vi "Multiple inputs.vi"() -> ()   [LabVIEW 2015]
doc: "This example VI shows how to convert string data elements to numeric elements so it can be graphed and displayed on an XY Graph."
uses:
  <instrlib>/Keithley 27XX/Keithley 27XX.lvlib
panel:
  in  "Column headers":string[](array[string])=["Time/s", "TH/Celsius", "TC/Celsius", "Delta V"]
  in  "Number of channels":i32=1
  in  "Pause/Continue":bool
  in  "stop":bool
  out "Numeric":i32
  out "concatenated string":string
  in  "file (use dialog)":path=path "C:/Users/Guest_2/Desktop/Zong Long/Data trial.txt"
  in  "Function (6: Temp)":u16(ring)=6 items=["DC Voltage", "AC Voltage", "DC Current", "AC Current", "Resistance", "Four-Wire Resistance", "Temperature (C)", "Frequency", "Period", "Continuity"]
  in  "Channel List (101)":string="101"
  in  "Serial Configuration":T1={"Baud Rate (9600)"=9600, "Flow Control (1: XON/XOFF)"=1, "Termination Char (0:CR)"=0} {"Termination Char (0:CR)" items=["CR", "LF", "CRLF (Do not use)", "LFCR (Do not use)"]; "Flow Control (1: XON/XOFF)" items=["None", "XON/XOFF", "RTS/CTS (2701 Only)", "XON/XOFF & RTS/CTS (2701 Only)"]; "Baud Rate (9600)" items=["300"=300, "600"=600, "1200"=1200, "2400"=2400, "4800"=4800, "9600"=9600, "19.2k"=19200, "38.4k (2701 Only)"=38400, "57.6k (2701 Only)"=57600, "115.2k (2701 Only)"=115200]}
  in  "VISA resource name":refnum<visa-resource-name>="GPIB0::19::INSTR"
  # "Remember to change the number of channels"
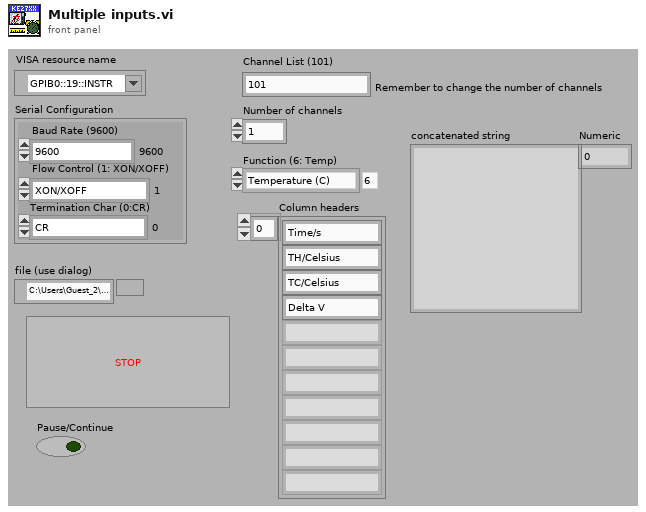
[diagram p1: front panel]
types:
  T1 = cluster{"Baud Rate (9600)":u32, "Flow Control (1: XON/XOFF)":u16, "Termination Char (0:CR)":u16}
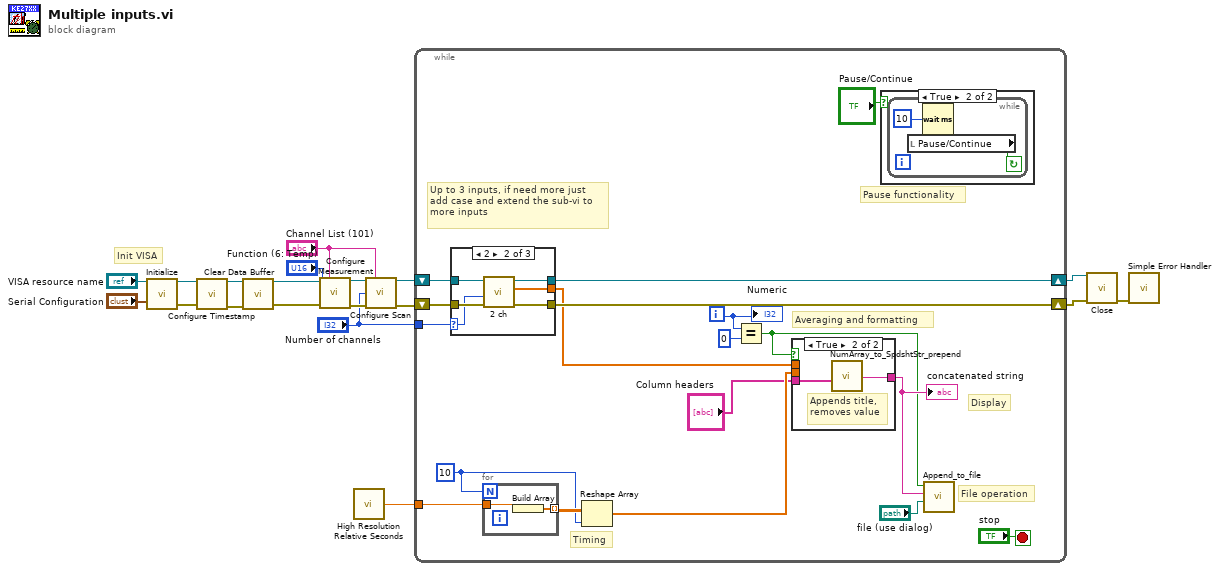
[diagram p0: block diagram]
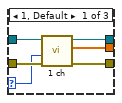
[diagram p2: hidden frame]
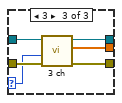
[diagram p3: hidden frame]
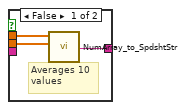
[diagram p5: hidden frame]
diagram:
  # "Init VISA"
  n1 = call <instrlib>:"Initialize.vi"("VISA resource name"="VISA resource name", "Serial Configuration"="Serial Configuration") -> ("VISA resource name out"=w16:refnum<visa-resource-name>, "error out"=w15:errorcluster)  [unwired: 12 in]
  n2 = call <instrlib>:"Configure Timestamp.vi"("VISA resource name"=w16, "error in (no error)"=w15) -> ("VISA resource name out"=w11:refnum<visa-resource-name>, "error out"=w10:errorcluster)  [unwired: 12 in]
  n3 = call <instrlib>:"Clear Data Buffer.vi"("VISA resource name"=w11, "error in (no error)"=w10) -> ("VISA resource name out"=w9:refnum<visa-resource-name>, "error out"=w12:errorcluster)  [unwired: 12 in]
  n4 = call <instrlib>:"Configure Measurement.vi"("VISA resource name"=w9, "Scan List (Empty)"="Channel List (101)", "Function (0: DC Voltage)"="Function (6: Temp)", "error in (no error)"=w12) -> ("VISA resource name out"=w8:refnum<visa-resource-name>, "error out"=w6:errorcluster)  [unwired: 10 in]
  n5 = call <vilib>:"High Resolution Relative Seconds.vi"() -> ("relative seconds"=w2:dbl)
  n6 = call <instrlib>:"Configure Scan.vi"("VISA resource name"=w8, "Channel List (101:110)"="Channel List (101)", "Sample Count (100)"="Number of channels", "error in (no error)"=w6) -> ("VISA resource name out"=w4:refnum<visa-resource-name>, "error out"=w3:errorcluster)  [unwired: 10 in]
  n7 = while {
    shift-right: [w36] -> w13
    shift-left: w4 -> [w35]
    shift-right: [w37] -> w14
    shift-left: w3 -> [w34]
    tunnel: w2 -> [w30]
    tunnel: "Number of channels" -> [w21]
    i -> [w24]
    stop <- "stop" stop-if-true
    w20 = 10 ("x")
    # "Timing"
    # "Up to 3 inputs, if need more just\nadd case and extend the sub-vi to\nmore inputs"
    # "Display"
    # "Averaging and formatting"
    # "File operation"
    # "Pause functionality"
    n8 = case shown="2" w21 {
      selector: w21 -> [w38 w44 w50]
      tunnel: [w41 w45 w51] -> w37
      tunnel: [w39 w47 w53] -> w36
      tunnel: w35 -> [w43 w49 w54]
      tunnel: w34 -> [w42 w48 w55]
      tunnel: [w40 w46 w52] -> w22
      frame 1, Default {
        n9 = call "1 ch.vi"("error out"=w42, "Number of channels"=w38, "VISA resource name out"=w43) -> ("error out 2"=w41:errorcluster, "output array"=w40:dbl[], "VISA resource name out 2"=w39:refnum<visa-resource-name>)  [unwired: 6 in]
      }
      frame 2 {
        n10 = call "2 ch.vi"("error out"=w48, "Number of channels"=w44, "VISA resource name out"=w49) -> ("error out 2"=w45:errorcluster, "output array"=w46:dbl[], "VISA resource name out 2"=w47:refnum<visa-resource-name>)  [unwired: 6 in]
      }
      frame 3 {
        n11 = call "3 ch.vi"("error out"=w55, "Number of channels"=w50, "VISA resource name out"=w54) -> ("error out 2"=w51:errorcluster, "output array"=w52:dbl[], "VISA resource name out 2"=w53:refnum<visa-resource-name>)  [unwired: 6 in]
      }
    }
    n12 = for {
      N: w20 -> [_]
      tunnel: w30 -> [w59]
      tunnel: [w58] -> w29 mode=indexing
      n13 = Build Array(w59) -> (w58:dbl[])
    }
    n14 = Reshape Array(w29, w20) -> (w28:dbl[])
    n15 = Equal?(x=w24, y=0) -> (x = y?=w26:bool)
    n16 = case shown="True" w26 {
      tunnel: w22 -> [w62 _]
      tunnel: w28 -> [w61 _]
      tunnel: [w60 w64] -> w32
      tunnel: "Column headers" -> [_ w63]
      frame False {
        # "Averages 10 \nvalues"
        n17 = call "NumArray_to_SpdshtStr.vi"("element 2"=w61, "element"=w62) -> ("concatenated string"=w60:string)  [unwired: 8 in, 1 out]
      }
      frame True {
        # "Appends title,\nremoves value"
        n18 = call "NumArray_to_SpdshtStr_prepend.vi"("Column headers"=w63) -> ("concatenated string"=w64:string)  [unwired: 10 in]
      }
    }
    "concatenated string" <- w32
    n19 = case shown="True" "Pause/Continue" {
      frame False {
      }
      frame True {
        n20 = while {
          stop <- w57 continue-if-true
          n21 = local read "Pause/Continue"() -> (w57:bool)
          n22 = Wait (ms)(milliseconds to wait=u32 10) -> ()  [unwired: 1 out]
        }
      }
    }
    n23 = call "Append_to_file.vi"("file path (use dialog)"="file (use dialog)", "text"=w32, "Boolean"=w26) -> ()  [unwired: 8 in, 1 out]
    "Numeric" <- w24
  }
  n24 = call <instrlib>:"Close.vi"("VISA resource name"=w13, "error in (no error)"=w14) -> ("error out"=w17:errorcluster)  [unwired: 13 in]
  n25 = call <vilib>:"Simple Error Handler.vi"("error in (no error)"=w17) -> ()  [unwired: 4 in, 5 out]
